vi "CSM Check - UserLog.vi"(8 "Matched Previous?":bool, 10 "Cross CSM Data (In)":T1={"Name (\"\" to Use UUID)"="", "Current State"="", "Arguments"="", "Source Message"={"‘State"="", "’Arguments"="", "’Error"={"status"=FALSE, "code"=0, "source"=""}}, "Source Module"="", "Complete(T)/Start(F)"=FALSE, "LogType"=enum."State Change", "Time Stamp"=timestamp(0 s since 1904-01-01)}, 11 "GlobalLogFilter.lvclass":refnum<class "LogFilter.lvclass">) -> (0 "Matched? (Dup)":bool, 2 "Cross CSM Data":T1={"Name (\"\" to Use UUID)"="", "Current State"="", "Arguments"="", "Source Message"={"‘State"="", "’Arguments"="", "’Error"={"status"=FALSE, "code"=0, "source"=""}}, "Source Module"="", "Complete(T)/Start(F)"=FALSE, "LogType"=enum."State Change", "Time Stamp"=timestamp(0 s since 1904-01-01)}, 3 "GlobalLogFilter.lvclass (Dup)":refnum<class "LogFilter.lvclass">)   [LabVIEW 2017, in "Communicable State Machine.lvlib" / "LogFilter.lvclass"]
doc: "### CSM Check - State.vi\n\n-- <b>Controls</b> --\n- <b>Matched Previous?</b>:\n- <b>Cross CSM Data (in)</b>:\n- <b>GlobalLogFilter.lvclass</b>:\n\n-- <b>Indicators</b> --\n- <b>Matched? (dup)</b>:\n- <b>Cross CSM Data</b>:\n- <b>GlobalLogFilter.lvclass (dup)</b>:"
uses:
  LogFilter.lvclass
  Typedef/_CSM_GlobalLog_MSG.ctl
  Typedef/_CSM_Response Source Message.ctl
  Typedef/_CSM_GlobalLog_MSG_TYPE.ctl
  LogFilter.lvclass/LogFilter.ctl
  Communicable State Machine.lvlib
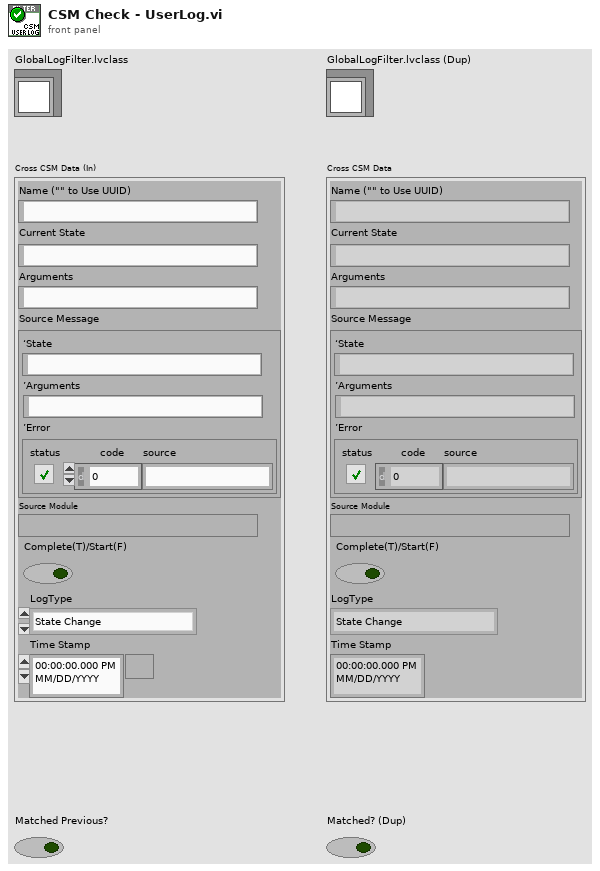
[diagram p1: front panel]
types:
  T1 = typedef "Communicable State Machine.lvlib/_CSM_GlobalLog_MSG.ctl" = cluster{"Name (\"\" to Use UUID)":string, "Current State":string, "Arguments":string, "Source Message":T2, "Source Module":string, "Complete(T)/Start(F)":bool, "LogType":T3, "Time Stamp":timestamp}
  T2 = typedef "Communicable State Machine.lvlib/_CSM_Response Source Message.ctl" = cluster{"‘State":string, "’Arguments":string, "’Error":errorcluster}
  T3 = typedef "Communicable State Machine.lvlib/_CSM_GlobalLog_MSG_TYPE.ctl" = enum16{"User Log", "State Change", "Status", "Interrupt", "Register", "Unregister", "Error Log", "Module Created", "Module Destroyed", "Async Message", "No-Rep Async Message", "Sync Message", "AsyncMsg Complete", "SyncMsg Complete"}
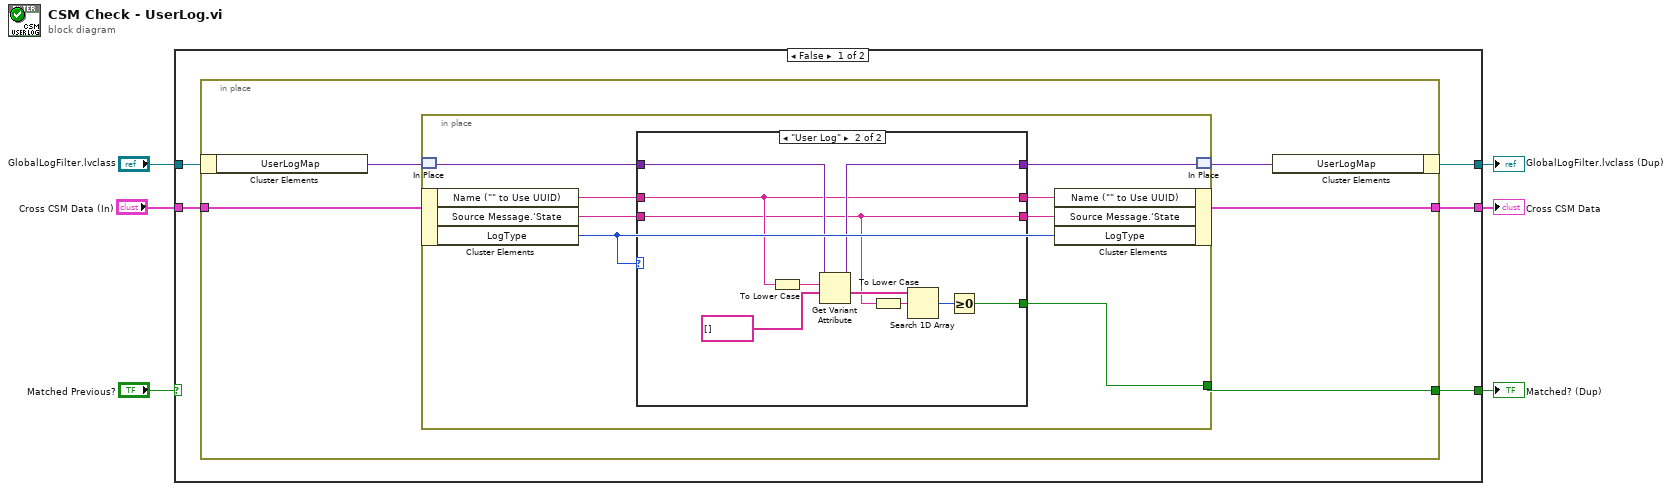
[diagram p0: block diagram]
diagram:
  n1 = case shown="False" "Matched Previous?" {
    selector: "Matched Previous?" -> [_ w39]
    tunnel: [w10 w40] -> w5
    tunnel: "Cross CSM Data (In)" -> [w11 w40]
    tunnel: [w9 w39] -> w3
    tunnel: [w7 w38] -> w2
    tunnel: "GlobalLogFilter.lvclass" -> [w8 w38]
    frame False {
      n2 = in-place {
        in-place-border: w11 -> [w16]
        in-place-border: [w15] -> w10
        in-place-border: [w14] -> w9
        n3 = in-place-cluster #1(w8) -> ("UserLogMap"=w13:variant)
        n4 = in-place {
          in-place-border: [w20] -> w14
          n5 = in-place-match #2(w13) -> (w24:variant)
          n6 = in-place-cluster #3(w16) -> ("Name (\"\" to Use UUID)"=w22:string, "Source Message.‘State"=w21:string, "LogType"=w19:T3)
          n7 = case shown="\"User Log\"" w19 {
            tunnel: w24 -> [w27 w37]
            tunnel: [w27 w36] -> w23
            tunnel: w22 -> [w25 w29]
            tunnel: w21 -> [w26 w28]
            tunnel: [_ w32] -> w20
            tunnel: [w25 w29] -> w18
            tunnel: [w26 w28] -> w17
            frame Default {
            }
            frame "User Log" {
              n8 = To Lower Case(string=w29) -> (all lower case string=w31:string)
              n9 = Get Variant Attribute(Variant=w37, name=w31, default value (empty Variant)=string[] []) -> (duplicate Variant=w36:variant, value=w34:string[])  [unwired: 1 in, 2 out]
              n10 = To Lower Case(string=w28) -> (all lower case string=w30:string)
              n11 = Search 1D Array(1D array=w34, element=w30) -> (index of element=w33:i32)  [unwired: 1 in]
              n12 = Greater Or Equal To 0?(x=w33) -> (x >= 0?=w32:bool)
            }
          }
          n13 = in-place-cluster #3("Name (\"\" to Use UUID)"=w18, "Source Message.‘State"=w17, "LogType"=w19) -> (w15:T1)
          n14 = in-place-match #2(w23) -> (w12:variant)
        }
        n15 = in-place-cluster #1("UserLogMap"=w12) -> (w7:refnum<class "LogFilter.lvclass">)
      }
    }
    frame True {
    }
  }
  "Cross CSM Data" <- w5
  "Matched? (Dup)" <- w3
  "GlobalLogFilter.lvclass (Dup)" <- w2
